vi "Result.vi"(8 "error in (no error)":errorcluster, 10 "Result":T1={"Name"="", "Message"="", "Description"="", "Status"=enum."Passed", "Result Type"=enum."Test Suite", "Execution Time"=0.0}, 11 "Icon Decorator In":refnum<class "Icon Decorator.lvclass">) -> (0 "error out":errorcluster)   [LabVIEW 2020, in "Icon Decorator.lvlib" / "Icon Decorator.lvclass"]
uses:
  Icon Decorator.lvclass
  Core/Result/Result.ctl
  Core/Result/Status.ctl
  Core/Result/Type.ctl
  Core/Result/Result.lvlib
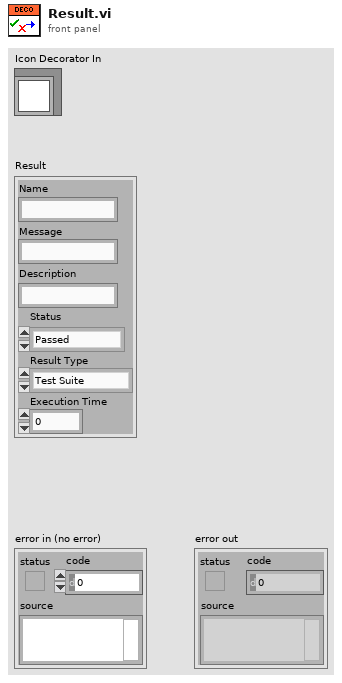
[diagram p1: front panel]
types:
  T1 = typedef "Result.lvlib/Result.ctl" = cluster{"Name":string, "Message":string, "Description":string, "Status":T2, "Result Type":T3, "Execution Time":dbl}
  T2 = typedef "Result.lvlib/Status.ctl" = enum16{"", "Passed", "Failed", "Error", "Skipped", "Setup Error", "Broken", "Teardown Error"}
  T3 = typedef "Result.lvlib/Type.ctl" = enum16{"Test Case", "Test Suite", "Test Run", "Pass", "Fail", "Skip", "Pass if", "Fail if", "Pass if Error", "Fail if Error", "Pass if Equal", "Fail if Equal"}
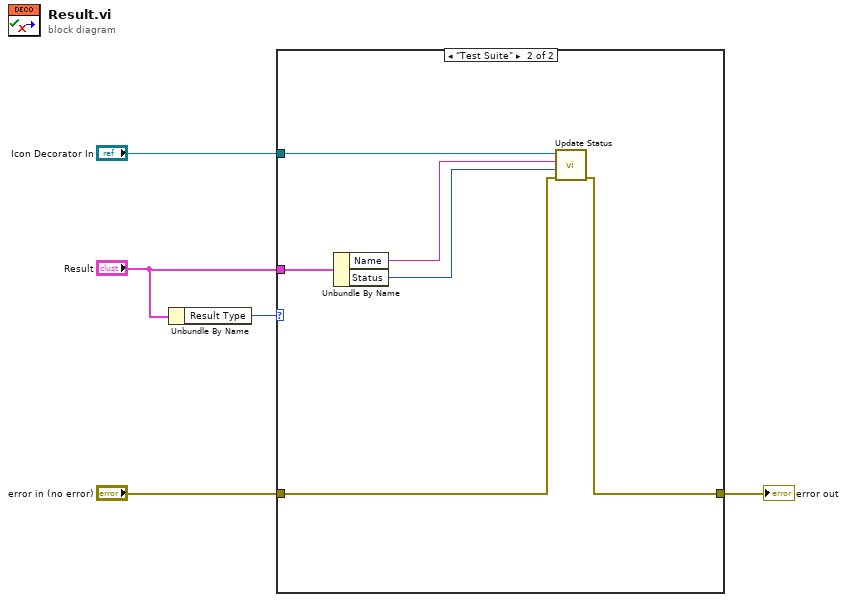
[diagram p0: block diagram]
diagram:
  n1 = Unbundle By Name("Result") -> ("Result Type"=w5:T3)
  n2 = case shown="\"Test Suite\"" w5 {
    tunnel: "Icon Decorator In" -> [_ w10]
    tunnel: "error in (no error)" -> [w6 w8]
    tunnel: "Result" -> [_ w12]
    tunnel: [w6 w7] -> w1
    frame Default {
    }
    frame "Test Suite" {
      n3 = Unbundle By Name(w12) -> ("Name"=w11:string, "Status"=w9:T2)
      n4 = call "Update Status.vi"("error in (no error)"=w8, "Status"=w9, "Case"=w11, "Icon Decorator In"=w10) -> ("error out"=w7:errorcluster)  [unwired: 7 in]
    }
  }
  "error out" <- w1
